vi "Open SystemLink Tag.vi"(6 "Connection Type":T2, 8 "error in (no error)":errorcluster, 9 "Path":string, 10 "Data Tag Type":T1, 11 "NI Skyline Configuration in":refnum<class "NI Skyline Configuration.lvclass">) -> (0 "error out":errorcluster, 3 "NI Skyline Tag out":refnum<class "NI Skyline Tag.lvclass">)   [LabVIEW 2015, in "SystemLink runtime.lvclass"]
doc: "Open SystemLink Tag Connection. \n\nResolves any template literals within the input path if required."
uses:
  SystemLink runtime.lvclass
  configuration/Connection Type.ctl
  <vilib>/Skyline/Configuration/Configuration_class/NI Skyline Configuration.lvclass
  configuration/Data Tag Type.ctl
  <vilib>/Skyline/Tag/Wrapper/Wrapper_class/NI Skyline Tag.lvclass
  <vilib>/Skyline/Configuration/Configuration HTTP_class/NI Skyline Configuration HTTP.lvclass
  <vilib>/Skyline/Configuration/Configuration AMQP_class/NI Skyline Configuration AMQP.lvclass
  <vilib>/Skyline/Tag/Wrapper/Wrapper HTTP_class/Open Tag HTTP.vi
  <vilib>/Skyline/Tag/Wrapper/Wrapper AMQP_class/Open Tag AMQP.vi
  configuration/SystemLink configuration.lvclass
  <vilib>/Skyline/Tag/Wrapper/Wrapper HTTP_class/NI Skyline Tag HTTP.lvclass
  <vilib>/Skyline/Tag/Wrapper/Wrapper AMQP_class/NI Skyline Tag AMQP.lvclass
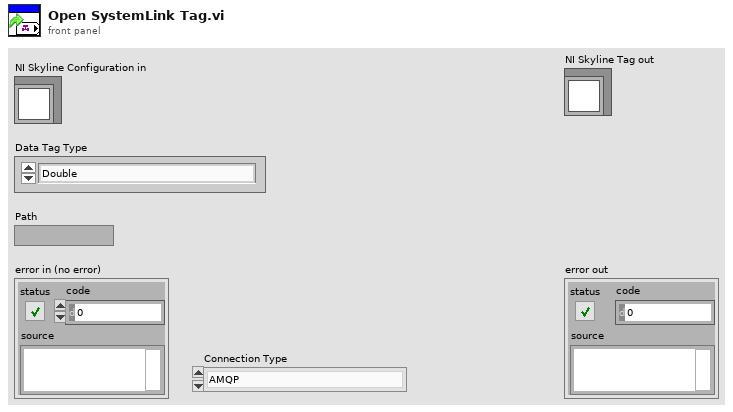
[diagram p1: front panel]
types:
  T1 = typedef "SystemLink configuration.lvclass/Data Tag Type.ctl" = enum16{"Double", "Single", "I32", "I16", "I8", "U64", "U32", "U16", "U8", "Boolean", "String", "Timestamp"}
  T2 = typedef "SystemLink configuration.lvclass/Connection Type.ctl" = enum16{"AMQP", "HTTP", "API Key (SystemLink Cloud)"}
  T3 = typedef "NI Skyline Tag.lvlib/DataType.ctl" = enum32{"Double", "I32", "String", "Boolean", "U64", "Timestamp"}
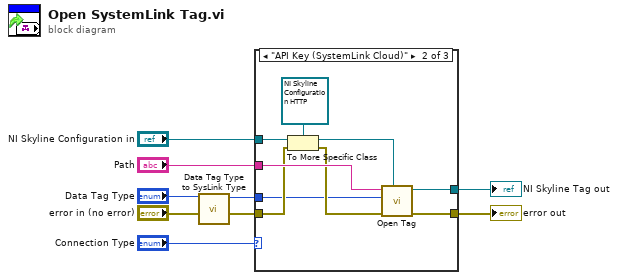
[diagram p0: block diagram]
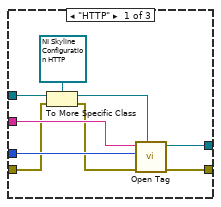
[diagram p2: hidden frame]
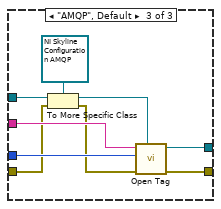
[diagram p3: hidden frame]
diagram:
  n1 = call "Data Tag Type to SysLink Type.vi"("Data Tag Type"="Data Tag Type") -> ("data type"=w3:T3)  [unwired: 10 in]
  n2 = case shown="\"API Key (SystemLink Cloud)\"" "Connection Type" {
    tunnel: "NI Skyline Configuration in" -> [w17 w26 w35]
    tunnel: w3 -> [w16 w18 w34]
    tunnel: "Path" -> [w15 w25 w33]
    tunnel: [w14 w24 w32] -> w7
    tunnel: "error in (no error)" -> [w11 w21 w29]
    tunnel: [w13 w23 w31] -> w6
    frame "HTTP" {
      n3 = To More Specific Class(target class=refnum<class "NI Skyline Configuration HTTP.lvclass"> refnum ("configuration"), reference=w17, error in=w11) -> (specific class reference=w12:refnum<class "NI Skyline Configuration HTTP.lvclass">, error out=w10:errorcluster)
      n4 = call-poly <vilib>:"Open Tag.vi"("configuration"=w12, "error in (no error)"=w10, "Data Type"=w16, "path"=w15) -> ("error out"=w14:errorcluster, "tag out"=w13:refnum<class "NI Skyline Tag.lvclass">)  [unwired: 6 in]
    }
    frame "API Key (SystemLink Cloud)" {
      n5 = To More Specific Class(target class=refnum<class "NI Skyline Configuration HTTP.lvclass"> refnum ("configuration"), reference=w26, error in=w21) -> (specific class reference=w22:refnum<class "NI Skyline Configuration HTTP.lvclass">, error out=w20:errorcluster)
      n6 = call-poly <vilib>:"Open Tag.vi"("configuration"=w22, "error in (no error)"=w20, "Data Type"=w18, "path"=w25) -> ("error out"=w24:errorcluster, "tag out"=w23:refnum<class "NI Skyline Tag.lvclass">)  [unwired: 6 in]
    }
    frame "AMQP", Default {
      n7 = To More Specific Class(target class=refnum<class "NI Skyline Configuration AMQP.lvclass"> refnum ("configuration"), reference=w35, error in=w29) -> (specific class reference=w30:refnum<class "NI Skyline Configuration AMQP.lvclass">, error out=w28:errorcluster)
      n8 = call-poly <vilib>:"Open Tag.vi"("configuration"=w30, "error in (no error)"=w28, "data type"=w34, "path"=w33) -> ("error out"=w32:errorcluster, "tag out"=w31:refnum<class "NI Skyline Tag.lvclass">)  [unwired: 6 in]
    }
  }
  "error out" <- w7
  "NI Skyline Tag out" <- w6
